vi "Init Communication.vi"() -> (0 "error out":errorcluster)   [LabVIEW 2017]
uses:
  Type Definitions/Controller Message.ctl
  Type Definitions/Controller States.ctl
  Type Definitions/Database Message.ctl
  Type Definitions/Database States.ctl
  Type Definitions/Display Console Message.ctl
  Type Definitions/Display Console States.ctl
  Type Definitions/GUI Message.ctl
  Type Definitions/Sensor Message.ctl
  Type Definitions/Sensor States.ctl
  Type Definitions/Queue FG Options.ctl
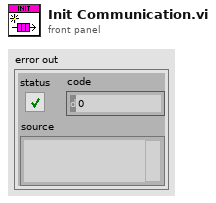
[diagram p1: front panel]
types:
  T1 = typedef "Queue FG Options.ctl" = enum16{"Set", "Get", "Read", "Write", "Destroy"}
  T2 = typedef "Sensor Message.ctl" = cluster{"Message Info":T3, "Message Data":variant}
  T3 = typedef "Sensor States.ctl" = enum16{"Initial", "Idle", "Shutdown"}
  T4 = typedef "GUI Message.ctl" = cluster{"Message Info":T5, "Message Data":variant}
  T5 = typedef "Controller States.ctl" = enum16{"Timeout", "Initial", "Login", "Idle", "Balance Inquiry", "Deposit", "Withdrawal", "Fast Cash", "Terminate", "Wait on Exit", "Shutdown", "Error Handler"}
  T6 = typedef "Display Console Message.ctl" = cluster{"Message Info":T7, "Message Data":variant}
  T7 = typedef "Display Console States.ctl" = enum16{"Timeout", "Initial", "Login", "Invalid Login", "Idle", "Balance Inquiry", "Deposit", "Withdrawal", "Fast Cash", "Withdrawal Failed", "Withdrawal Complete", "Terminate", "Shutdown"}
  T8 = typedef "Database Message.ctl" = cluster{"Message Info":T9, "Message Data":variant}
  T9 = typedef "Database States.ctl" = enum16{"Initial", "Verify", "Balance Inquiry", "Deposit", "Withdrawal", "Fast Cash", "Terminate", "Shutdown"}
  T10 = typedef "Controller Message.ctl" = cluster{"Message Info":T5, "Message Data":variant}
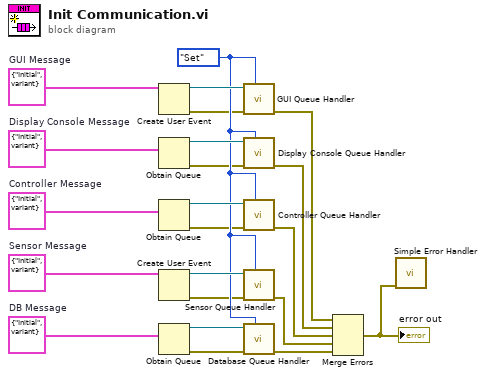
[diagram p0: block diagram]
diagram:
  w12 = Queue_FG_Options."Set" ("Action")
  w18 = T2 {"Message Info"=enum."Initial", "Message Data"=variant}  # Sensor Message
  w19 = T4 {"Message Info"=enum."Initial", "Message Data"=variant}  # GUI Message
  w20 = T6 {"Message Info"=enum."Initial", "Message Data"=variant}  # Display Console Message
  w21 = T8 {"Message Info"=enum."Initial", "Message Data"=variant}  # DB Message
  w22 = T10 {"Message Info"=enum."Initial", "Message Data"=variant}  # Controller Message
  n1 = Create User Event(user event datatype=w19) -> (user event=w13:refnum<user-event>, error out=w2:errorcluster)  [unwired: 1 in]
  n2 = Obtain Queue(element data type=w20) -> (queue out=w14:refnum<queue>, error out=w3:errorcluster)  [unwired: 4 in, 1 out]
  n3 = Obtain Queue(element data type=w22) -> (queue out=w15:refnum<queue>, error out=w4:errorcluster)  [unwired: 4 in, 1 out]
  n4 = Create User Event(user event datatype=w18) -> (user event=w17:refnum<user-event>, error out=w5:errorcluster)  [unwired: 1 in]
  n5 = Obtain Queue(element data type=w21) -> (queue out=w16:refnum<queue>, error out=w6:errorcluster)  [unwired: 4 in, 1 out]
  n6 = call "GUI Queue Handler.vi"("Action"=w12, "error in (no error)"=w2, "User event in"=w13) -> ("error out"=w11:errorcluster)  [unwired: 5 in, 3 out]
  n7 = call "Display Console Queue Handler.vi"("Action"=w12, "error in (no error)"=w3, "Queue in"=w14) -> ("error out"=w9:errorcluster)  [unwired: 6 in, 2 out]
  n8 = call "Controller Queue Handler.vi"("Action"=w12, "error in (no error)"=w4, "Queue in"=w15) -> ("error out"=w8:errorcluster)  [unwired: 6 in, 2 out]
  n9 = call "Sensor Queue Handler.vi"("Action"=w12, "error in (no error)"=w5, "User event in"=w17) -> ("error out"=w7:errorcluster)  [unwired: 5 in, 3 out]
  n10 = call "Database Queue Handler.vi"("Action"=w12, "error in (no error)"=w6, "Queue in"=w16) -> ("error out"=w10:errorcluster)  [unwired: 6 in, 2 out]
  n11 = Merge Errors(w11, w9, w8, w7, w10) -> (w1:errorcluster)
  "error out" <- w1
  n12 = call <vilib>:"Simple Error Handler.vi"("error in (no error)"=w1) -> ()  [unwired: 4 in, 5 out]
